vi "Set_Hi-Tec_server.vi"(4 "Client Name":string, 6 "Strength (% by volume)":dbl min=0.0 max=5.0 format="%.3f", 7 "Carrier_2 Q (l/min)":dbl=20.0 format="%.2f", 8 "Carrier_1 Q (l/min)":dbl=20.0 format="%.2f", 9 "Mode":enum16{"Control Hi-Tec", "Check Hi-Tec Demands"}(ring)) -> (0 "Flowrates (kg/min)":dbl[](array[numeric]) format="%.2f", 1 "Comment":string)   [LabVIEW 2015]
uses:
  ADAM Client/Sub VIs/ADAM Controls/Ch_description_ADAM.ctl
  ADAM Client/Sub VIs/ADAM Controls/Module_type_ADAM.ctl
  ADAM Client/Sub VIs/ADAM Controls/Function_ADAM.ctl
  ADAM Client/Sub VIs/ADAM Controls/Channel_State.ctl
  ADAM Client/Sub VIs/ADAM Controls/Calib_type_ADAM.ctl
  ADAM Client/Sub VIs/ADAM Controls/Address.ctl
  ADAM Client/Sub VIs/ADAM Controls/Update_scan_value.ctl
  Anemometry/Anemometry Sub Vis/Globals/Gas_management_global.vi
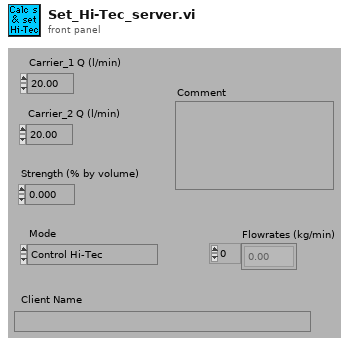
[diagram p1: front panel]
types:
  T1 = enum16{"Append to Global", "Read Global then Clear"}
  T2 = typedef "Calib_type_ADAM.ctl" = enum16{"Raw", "Bx + A", "Cx^2 + Bx + A", "Dx^3 + Cx^2 + Bx + A", "In Band", "Hi-Tec Q", "Hi-Tec M_dot", "Text"}
  T3 = typedef "Module_type_ADAM.ctl" = string
  T4 = typedef "Ch_description_ADAM.ctl" = cluster{"Ch Name":string, "Type":T3, "Function":T5, "Ch State":T6, "Calibration type":T2, "A":dbl, "B":dbl, "C":dbl, "D":dbl, "Comments":string, "Address":T7, "String":string, "Duty":u16}
  T5 = typedef "Function_ADAM.ctl" = enum16{"Analogue Input", "Digital Input", "Event counter", "Event rate", "Analogue Output", "Digital Output", "Relay Output"}
  T6 = typedef "Channel_State.ctl" = enum16{"On", "Off", "Always On", "Always Off"}
  T7 = typedef "Address.ctl" = cluster{"Main":i32, "Ch.":i32, "Sub":i32, "Port Name":string}
  T8 = typedef "Update_scan_value.ctl" = cluster{"Channel Name":string, "New Value":dbl}
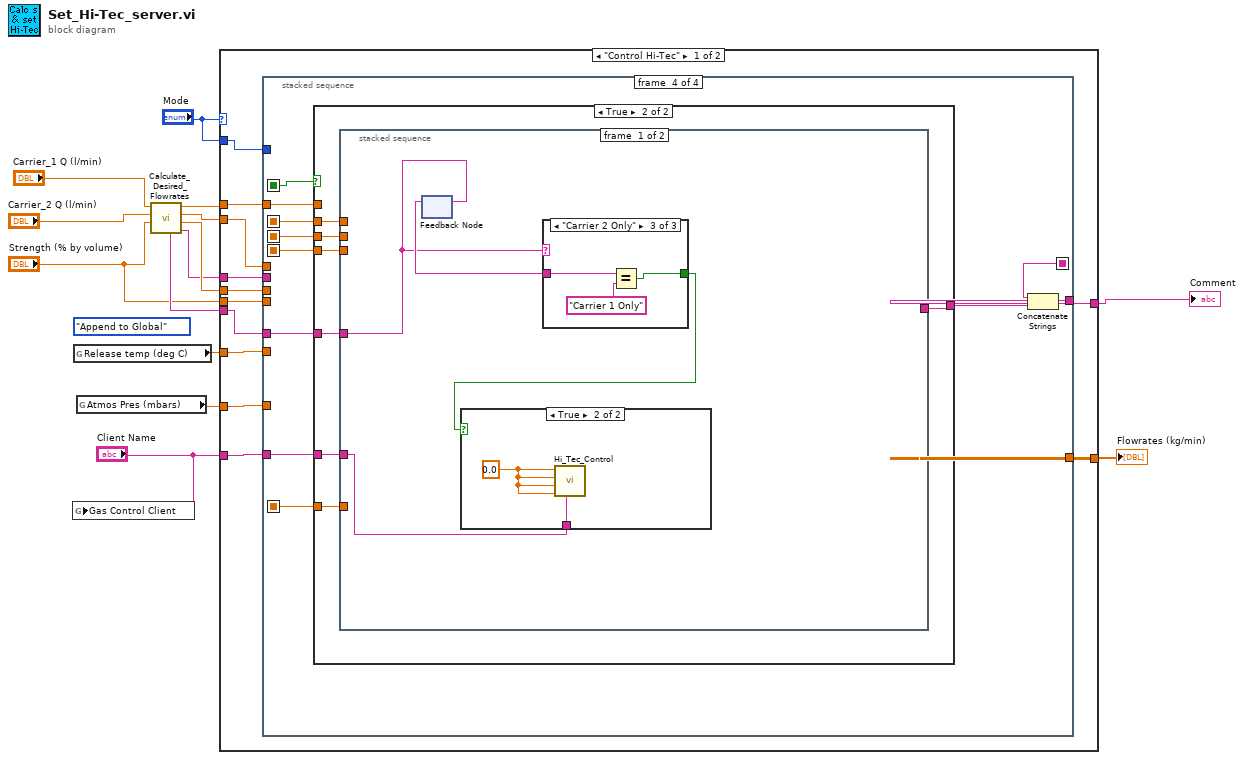
[diagram p0: block diagram]
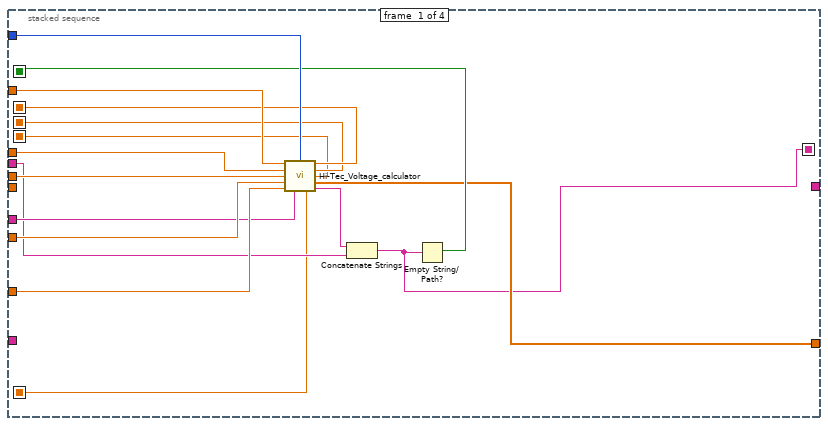
[diagram p2: hidden frame]
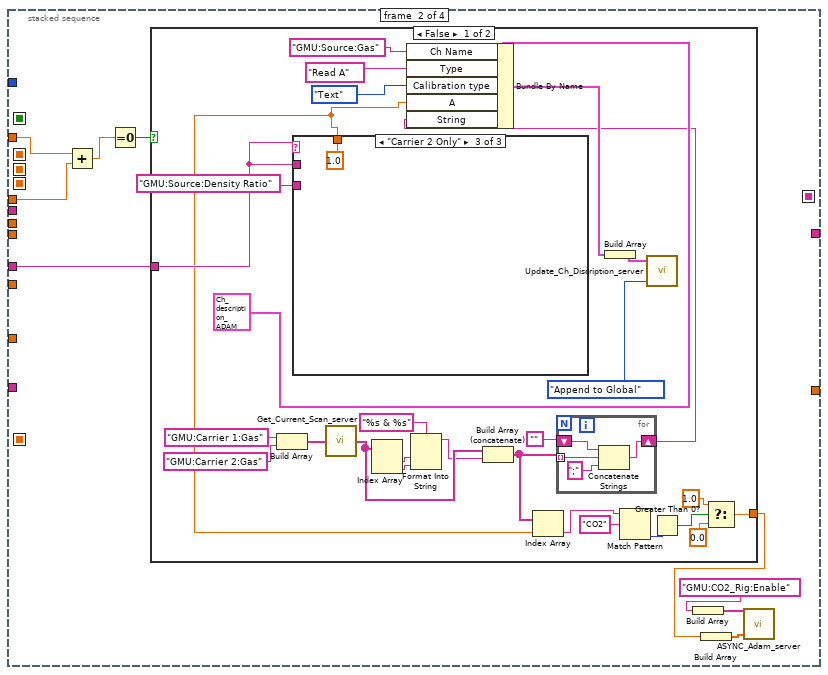
[diagram p3: hidden frame]
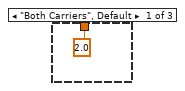
[diagram p4: hidden frame]
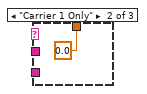
[diagram p5: hidden frame]
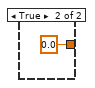
[diagram p6: hidden frame]
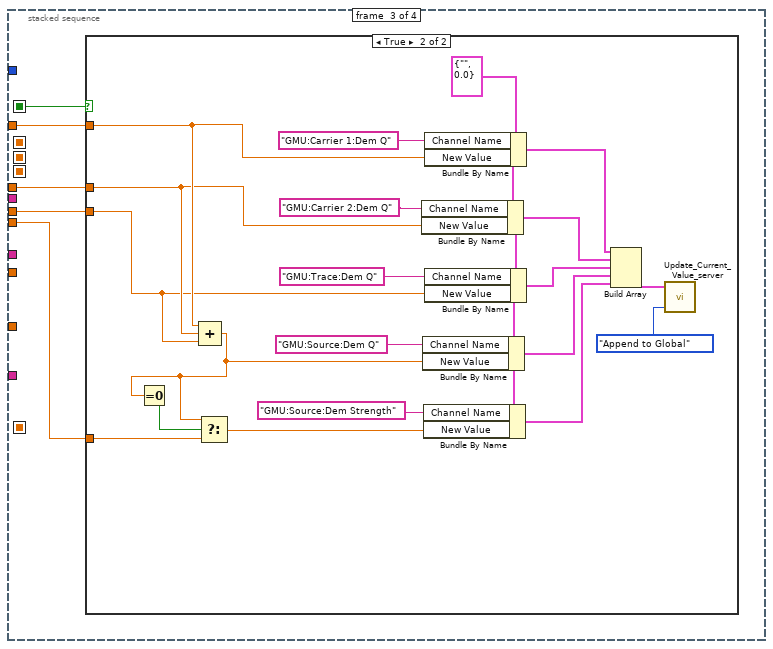
[diagram p7: hidden frame]
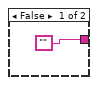
[diagram p9: hidden frame]
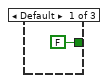
[diagram p10: hidden frame]
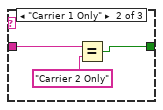
[diagram p11: hidden frame]
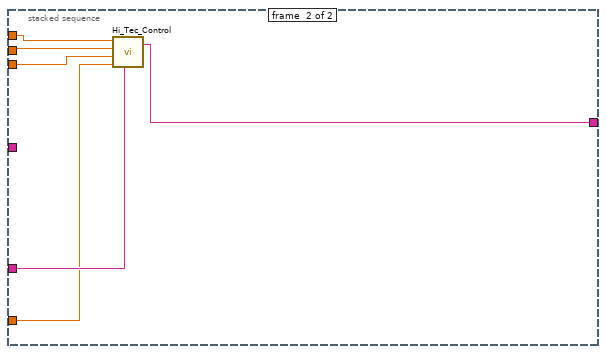
[diagram p13: hidden frame]
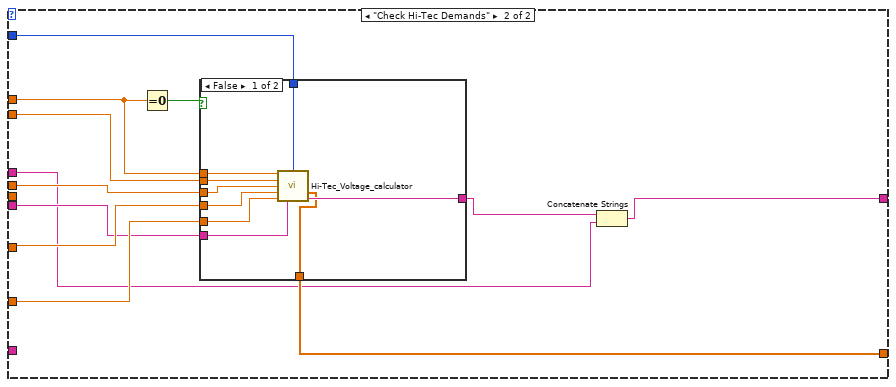
[diagram p14: hidden frame]
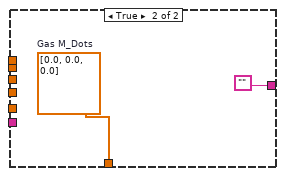
[diagram p15: hidden frame]
diagram:
  (unwired) T1."Append to Global" ("Mode")
  n1 = global write "Gas_management_global.vi" "Gas Control Client"("Client Name") -> ()
  n2 = global read "Gas_management_global.vi" "Release temp (deg C)"() -> (w13:dbl)
  n3 = global read "Gas_management_global.vi" "Atmos Pres (mbars)"() -> (w14:dbl)
  n4 = call "Calculate_Desired_Flowrates.vi"("Strength (% by volume)"="Strength (% by volume)", "Carrier_2 Q (l/min)"="Carrier_2 Q (l/min)", "Carrier_1 Q (l/min)"="Carrier_1 Q (l/min)") -> ("Error Message"=w2:string, "Trace Q l/min"=w5:dbl, "Carrier 2 l/min"=w6:dbl, "Carrier 1 l/min"=w7:dbl, "Carrier Info"=w4:string)  [unwired: 3 in]
  n5 = case shown="\"Control Hi-Tec\"" "Mode" {
    tunnel: w7 -> [w26 w160]
    tunnel: w13 -> [w25 w162]
    tunnel: w14 -> [w24 w161]
    tunnel: [w23 w152] -> w1
    tunnel: [w22 w158] -> w12
    tunnel: "Mode" -> [w21 w157]
    tunnel: "Client Name" -> [w20 _]
    tunnel: w6 -> [w19 w156]
    tunnel: w5 -> [w18 w155]
    tunnel: w4 -> [w17 w154]
    tunnel: "Strength (% by volume)" -> [w16 _]
    tunnel: w2 -> [w15 w151]
    frame "Control Hi-Tec" {
      n6 = stacked-sequence {
        seq-local: [w37 _ _ _] -> [_ _ w92 w119]
        seq-local: [w36 _ _ _] -> [_ _ _ w123]
        seq-local: [w35 _ _ _] -> [_ _ _ w122]
        seq-local: [w34 _ _ _] -> [_ _ _ w121]
        seq-local: [w28 _ _ _] -> [_ _ _ w116]
        seq-local: [w27 _ _ _] -> [_ _ _ w113]
        tunnel: w19 -> [w40 w43 w90 _]
        tunnel: w26 -> [w39 w44 w91 w118]
        tunnel: w25 -> [w42 _ _ _]
        tunnel: w24 -> [w41 _ _ _]
        tunnel: [_ _ _ w117] -> w23
        tunnel: [w31 _ _ _] -> w22
        tunnel: w21 -> [w38 _ _ _]
        tunnel: w20 -> [_ _ _ w120]
        tunnel: w18 -> [w33 _ w89 _]
        tunnel: w17 -> [w32 w46 _ w114]
        tunnel: w16 -> [_ _ w88 _]
        tunnel: w15 -> [w29 _ _ _]
        frame #0 {
          n7 = call "Hi-Tec_Voltage_calculator.vi"("Carrier_1 Q (l/min)"=w39, "Mode"=w38, "Carrier_2 Q (l/min)"=w40, "Trace Q (l/min)"=w33, "Release temp (deg C)"=w42, "Atmos Pres (mbars)"=w41, "Carrier Info"=w32) -> ("Carrier 1 Voltage"=w36:dbl, "Carrier 2 Voltage"=w35:dbl, "Trace Voltage"=w34:dbl, "Flowrates (kg/min)"=w31:dbl[], "Trace_2 Voltage"=w27:dbl, "Error Comments"=w30:string)  [unwired: 2 in, 1 out]
          n8 = Concatenate Strings(w30, w29) -> (w28:string)
          n9 = Empty String/Path?(string/path=w28) -> (empty?=w37:bool)
        }
        frame #1 {
          n10 = Add(x=w44, y=w43) -> (x+y=w45:dbl)
          n11 = Equal To 0?(x=w45) -> (x = 0?=w51:bool)
          n12 = case shown="False" w51 {
            tunnel: w46 -> [w77 _]
            tunnel: [w52 0.0 ("f")] -> w47
            frame False {
              n13 = Build Array("GMU:Carrier 1:Gas", "GMU:Carrier 2:Gas") -> (w76:string[])
              n14 = case shown="\"Carrier 2 Only\"" w77 {
                tunnel: "GMU:Source:Density Ratio" -> [_ _ _]
                tunnel: w77 -> [_ _ _]
                tunnel: [2.0 ("A") 0.0 ("A") 1.0 ("A")] -> w59
                frame "Both Carriers", Default {
                }
                frame "Carrier 1 Only" {
                }
                frame "Carrier 2 Only" {
                }
              }
              n15 = call "Get_Current_Scan_server.vi"("Desired Channels"=w76) -> ("String values"=w65:string[])  [unwired: 2 out]
              n16 = Index Array(array=w65) -> (element #1=w68:string, element #2=w67:string)  [unwired: 2 in]
              n17 = Format Into String(format string="%s & %s", w68, w67) -> (resulting string=w64:string)  [unwired: 2 in, 1 out]
              n18 = Build Array (concatenate)(w65, w64) -> (w60:string[])
              n19 = Index Array(array=w60, index=w59) -> (element=w57:string)
              n20 = for {
                shift-right: [w83] -> w61
                shift-left: "" -> [w82]
                tunnel: w60 -> [w81] mode=indexing
                n21 = Concatenate Strings(w82, w81, ";" ("string")) -> (w83:string)
              }
              n22 = Bundle By Name(cluster=T4 {"Ch Name"="", "Type"="", "Function"=enum."Analogue Input", "Ch State"=enum."On", "Calibration type"=enum."Raw", "A"=0.0, "B"=0.0, "C"=0.0, "D"=0.0, "Comments"="", "Address"={"Main"=0, "Ch."=0, "Sub"=0, "Port Name"=""}, "String"="", "Duty"=65535} ("Ch Discription"), "Ch Name"="GMU:Source:Gas", "Type"=T3 "Read A", "Calibration type"=Calib_type_ADAM."Text", "A"=w59, "String"=w61) -> (w70:T4)
              n23 = Build Array(w70) -> (w78:T4[])
              n24 = Match Pattern(string=w57, regular expression="CO2") -> (offset past match=w56:i32)  [unwired: 1 in, 3 out]
              n25 = call "Update_Ch_Discription_server.vi"("Mode"=T1."Append to Global", "Channels to update In"=w78) -> ()  [unwired: 1 in, 1 out]
              n26 = Greater Than 0?(x=w56) -> (x > 0?=w55:bool)
              n27 = Select(t=1.0, s=w55, f=0.0) -> (s? t:f=w52:dbl)
            }
            frame True {
            }
          }
          n28 = Build Array("GMU:CO2_Rig:Enable") -> (w49:string[])
          n29 = Build Array(w47) -> (w50:dbl[])
          n30 = call "ASYNC_Adam_server.vi"("Values"=w50, "Channel Names"=w49) -> ()  [unwired: 1 in, 3 out]
        }
        frame #2 {
          n31 = case shown="True" w92 {
            tunnel: w91 -> [_ w103]
            tunnel: w90 -> [_ w102]
            tunnel: w89 -> [_ w101]
            tunnel: w88 -> [_ w99]
            frame False {
            }
            frame True {
              w98 = T8 {"Channel Name"="", "New Value"=0.0} ("Update Scan Value Cluster")
              n32 = Compound Arithmetic op=ADD(w103, w102, w101) -> (w100:dbl)
              n33 = Equal To 0?(x=w100) -> (x = 0?=w108:bool)
              n34 = Select(t=w100, s=w108, f=w99) -> (s? t:f=w107:dbl)
              n35 = Bundle By Name(cluster=w98, "Channel Name"="GMU:Carrier 2:Dem Q", "New Value"=w102) -> (w96:T8)
              n36 = Bundle By Name(cluster=w98, "Channel Name"="GMU:Source:Dem Q", "New Value"=w100) -> (w94:T8)
              n37 = Bundle By Name(cluster=w98, "Channel Name"="GMU:Source:Dem Strength", "New Value"=w107) -> (w93:T8)
              n38 = Bundle By Name(cluster=w98, "Channel Name"="GMU:Carrier 1:Dem Q", "New Value"=w103) -> (w97:T8)
              n39 = Bundle By Name(cluster=w98, "Channel Name"="GMU:Trace:Dem Q", "New Value"=w101) -> (w95:T8)
              n40 = Build Array(w97, w96, w95, w94, w93) -> (w110:T8[])
              n41 = call "Update_Current_Value_server.vi"("Mode"=T1."Append to Global", "Update array in"=w110) -> ()  [unwired: 1 in, 1 out]
            }
          }
        }
        frame #3 {
          n42 = case shown="True" w119 {
            tunnel: w123 -> [_ w131]
            tunnel: w122 -> [_ w130]
            tunnel: w121 -> [_ w129]
            tunnel: w120 -> [_ w128]
            tunnel: w118 -> [_ _]
            tunnel: ["" w127] -> w115
            tunnel: w114 -> [_ w126]
            tunnel: w113 -> [_ w125]
            frame False {
            }
            frame True {
              n43 = stacked-sequence {
                tunnel: w131 -> [_ w150]
                tunnel: w130 -> [_ w149]
                tunnel: w129 -> [_ w148]
                tunnel: w128 -> [w135 w147]
                tunnel: [_ w146] -> w127
                tunnel: w126 -> [w132 _]
                tunnel: w125 -> [_ w145]
                frame #0 {
                  n44 = feedback-in #1(w132) -> ()
                  n45 = feedback #1() -> (w134:string)  [unwired: 1 in]
                  n46 = case shown="\"Carrier 2 Only\"" w132 {
                    tunnel: w134 -> [_ w139 w142]
                    tunnel: [FALSE w137 w140] -> w133
                    frame Default {
                    }
                    frame "Carrier 1 Only" {
                      n47 = Equal?(x=w139, y="Carrier 2 Only") -> (x = y?=w137:bool)
                    }
                    frame "Carrier 2 Only" {
                      n48 = Equal?(x=w142, y="Carrier 1 Only") -> (x = y?=w140:bool)
                    }
                  }
                  n49 = case shown="True" w133 {
                    tunnel: w135 -> [_ w144]
                    frame False {
                    }
                    frame True {
                      w143 = 0.0 ("Carrier 1 Voltage")
                      n50 = call "Hi_Tec_Control.vi"("Carrier 1 Voltage"=w143, "Carrier 2 Voltage"=w143, "Trace Voltage"=w143, "Trace_2 Voltage"=w143, "Client Name"=w144) -> ()  [unwired: 2 out]
                    }
                  }
                }
                frame #1 {
                  n51 = call "Hi_Tec_Control.vi"("Carrier 1 Voltage"=w150, "Carrier 2 Voltage"=w149, "Trace Voltage"=w148, "Trace_2 Voltage"=w145, "Client Name"=w147) -> ("Scan Comments"=w146:string)  [unwired: 1 out]
                }
              }
            }
          }
          n52 = Concatenate Strings(w116, w115) -> (w117:string)
        }
      }
    }
    frame "Check Hi-Tec Demands" {
      n53 = Equal To 0?(x=w160) -> (x = 0?=w159:bool)
      n54 = case shown="False" w159 {
        tunnel: w156 -> [w171 _]
        tunnel: w162 -> [w170 _]
        tunnel: w161 -> [w169 _]
        tunnel: [w168 ""] -> w153
        tunnel: w160 -> [w167 _]
        tunnel: [w164 w172] -> w158
        tunnel: w157 -> [w166 _]
        tunnel: w155 -> [w165 _]
        tunnel: w154 -> [w163 _]
        frame False {
          n55 = call "Hi-Tec_Voltage_calculator.vi"("Carrier_1 Q (l/min)"=w167, "Mode"=w166, "Carrier_2 Q (l/min)"=w171, "Trace Q (l/min)"=w165, "Release temp (deg C)"=w170, "Atmos Pres (mbars)"=w169, "Carrier Info"=w163) -> ("Flowrates (kg/min)"=w164:dbl[], "Error Comments"=w168:string)  [unwired: 1 in, 6 out]
        }
        frame True {
          w172 = dbl[] [0.0, 0.0, 0.0]  # Gas M_Dots
        }
      }
      n56 = Concatenate Strings(w153, w151) -> (w152:string)
    }
  }
  "Comment" <- w1
  "Flowrates (kg/min)" <- w12
